vi "hari_Challenge1.vi"   [LabVIEW 2014, in "Malladi_Achanta_5_LEGORobotics_11-29-16.lvrbt"]
uses:
  Malladi_Achanta_5_LEGORobotics_11-29-16.lvrbt
  <vilib>/NXT/Block Support/NXT_InputPort.ctl
  <vilib>/NXT/Block Support/NXT_OutputPort.ctl
  <vilib>/NXT/Dual Mode Library/Sensors/Sonar_cm.vi
  <vilib>/NXT/NXTIO Xnodes/NXTIONodeSubVIs/NXTMoveMotors.vi
  <vilib>/NXT/Dual Mode Library/Waits/Wait_Num.vi
  <vilib>/NXT/NXTIO Xnodes/NXTIONodeSubVIs/LEGOStopAllMotors.vi
  <vilib>/NXT/NXTIO Xnodes/AddressXNode/NXTIOAddress.xnode
  <vilib>/NXT/NXTIO Xnodes/NXTIOXNode/NXTIO.xnode
  <vilib>/NXT/Subs/LVHSConnector.ctl
  <vilib>/NXT/LegoClasses/BrickReference/BrickReference.lvclass
types:
  T1 = typedef "NXT_OutputPort.ctl" = u8
  T2 = typedef "NXT_InputPort.ctl" = u32
  T3 = typedef "LVHSConnector.ctl" = refnum<class "BrickReference.lvclass">
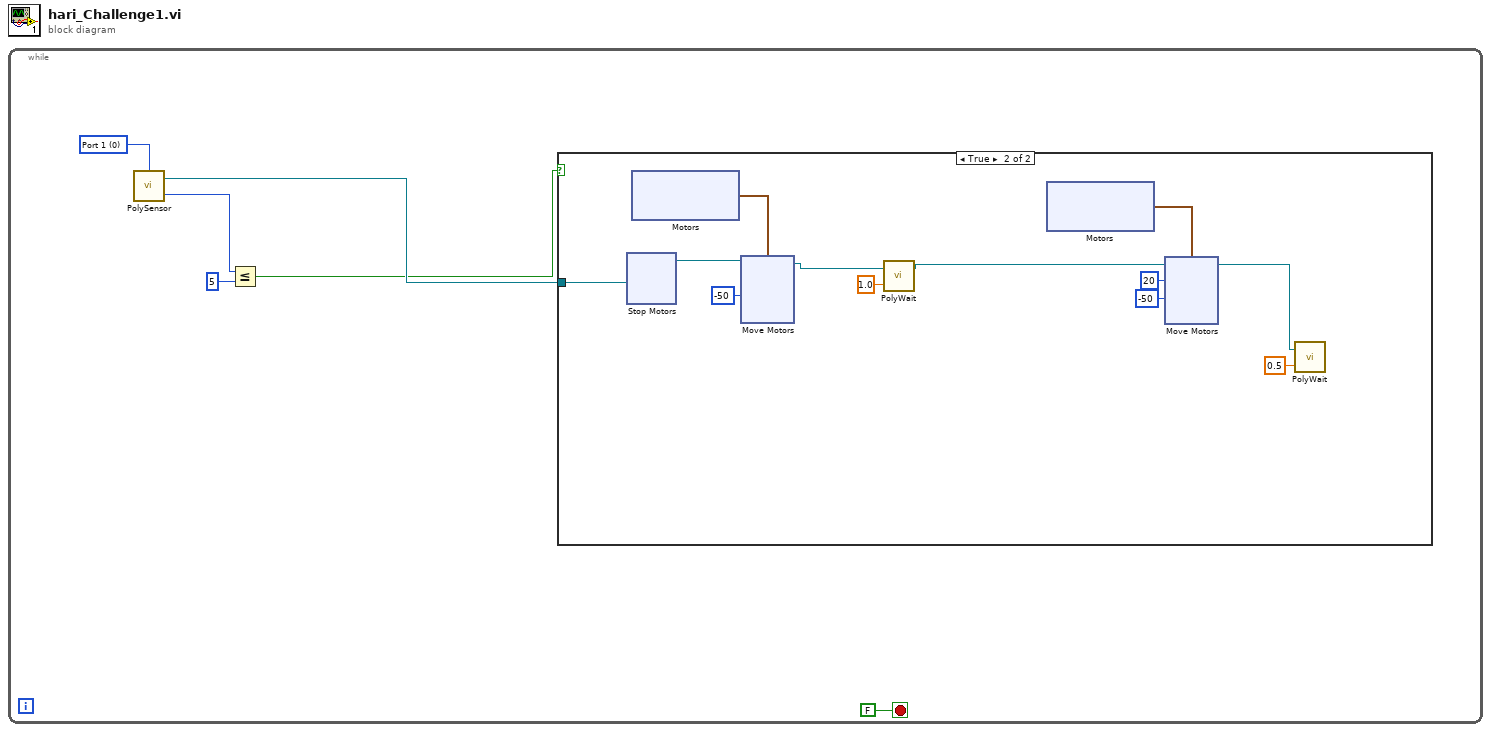
[diagram p0: block diagram]
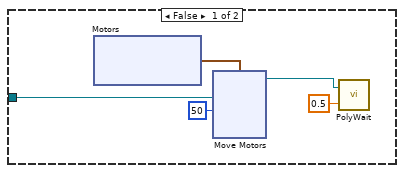
[diagram p2: hidden frame]
diagram:
  n1 = while {
    stop <- FALSE stop-if-true
    w2 = T2 0 items=["Port 1", "Port 2", "Port 3", "Port 4"] ("Port (Port 4)")
    n2 = call-poly <vilib>:"PolySensor.vi"("Port (Port 4)"=w2) -> ("Distance (cm)"=w4:i16, "NXT/EV3"=w5:T3)  [unwired: 2 in]
    n3 = Less Or Equal?(x=w4, y=i16 5) -> (x <= y?=w1:bool)
    n4 = case shown="True" w1 {
      tunnel: w5 -> [w10 w32]
      frame False {
        n5 = xnode "Motors"() -> ("Motor"=w11:cluster{"Port":T1, "Port":T1})
        n6 = xnode "Move Motors"("Power/Speed 2"=i8 50, "Motors"=w11, "NXT/EV3"=w10) -> ("NXT/EV3"=w8:T3)  [unwired: 1 in]
        n7 = call-poly <vilib>:"PolyWait.vi"("Time (1 sec)"=sgl 0.5, "NXT/EV3"=w8) -> ()  [unwired: 2 in, 1 out]
      }
      frame True {
        n8 = xnode "Stop Motors"("NXT/EV3"=w32) -> ("NXT/EV3"=w27:T3)  [unwired: 1 in]
        n9 = xnode "Motors"() -> ("Motor"=w31:cluster{"Port":T1, "Port":T1})
        n10 = xnode "Move Motors"("Power/Speed 2"=i8 -50, "Motors"=w31, "NXT/EV3"=w27) -> ("NXT/EV3"=w28:T3)  [unwired: 1 in]
        n11 = call-poly <vilib>:"PolyWait.vi"("Time (1 sec)"=sgl 1.0, "NXT/EV3"=w28) -> ("NXT/EV3"=w26:T3)  [unwired: 2 in]
        n12 = xnode "Motors"() -> ("Motor"=w25:cluster{"Port":T1, "Port":T1})
        n13 = xnode "Move Motors"("Power/Speed 2"=i8 -50, "Power/Speed 1"=i8 20, "Motors"=w25, "NXT/EV3"=w26) -> ("NXT/EV3"=w22:T3)
        n14 = call-poly <vilib>:"PolyWait.vi"("Time (1 sec)"=sgl 0.5, "NXT/EV3"=w22) -> ()  [unwired: 2 in, 1 out]
      }
    }
  }
